vi "Close Manager Refs.vi"(8 "error in (no error)":errorcluster, 11 "teststand-api in":refnum<class "teststand-api.lvclass">) -> (0 "error out":errorcluster, 3 "teststand-api out":refnum<class "teststand-api.lvclass">)   [LabVIEW 2014, in "teststand-api.lvlib" / "teststand-api.lvclass"]
uses:
  teststand-api.lvclass
  teststand-api.lvclass/teststand-api.ctl
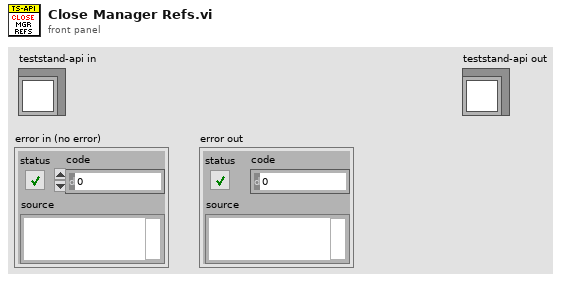
[diagram p1: front panel]
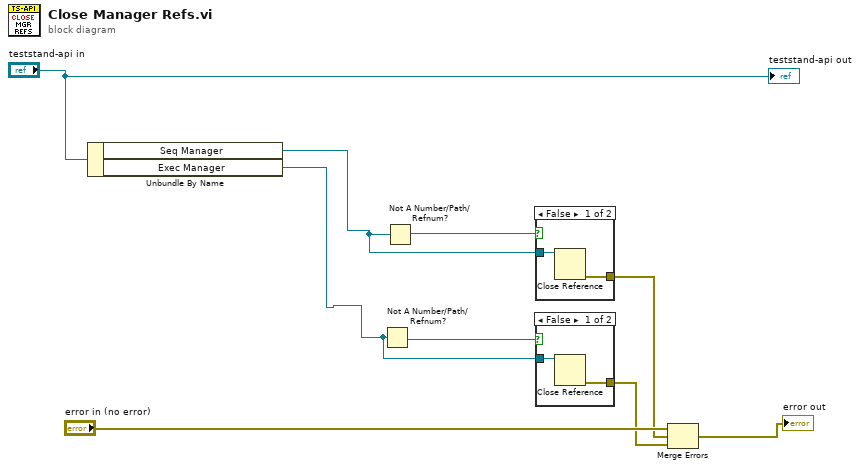
[diagram p0: block diagram]
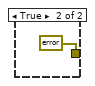
[diagram p2: hidden frame]
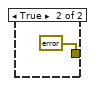
[diagram p3: hidden frame]
diagram:
  n1 = Unbundle By Name("teststand-api in") -> ("Seq Manager"=w5:refnum<k7>, "Exec Manager"=w3:refnum<k7>)
  n2 = Not A Number/Path/Refnum?(number/path/refnum=w3) -> (NaN/Path/Refnum?=w4:bool)
  n3 = Not A Number/Path/Refnum?(number/path/refnum=w5) -> (NaN/Path/Refnum?=w6:bool)
  n4 = case shown="False" w6 {
    tunnel: [w11 errorcluster {"status"=FALSE, "code"=0, "source"=""} ("error out")] -> w2
    tunnel: w5 -> [w10 _]
    frame False {
      n5 = Close Reference(reference=w10) -> (error out=w11:errorcluster)  [unwired: 1 in]
    }
    frame True {
    }
  }
  n6 = case shown="False" w4 {
    tunnel: [w14 errorcluster {"status"=FALSE, "code"=0, "source"=""} ("error out")] -> w1
    tunnel: w3 -> [w13 _]
    frame False {
      n7 = Close Reference(reference=w13) -> (error out=w14:errorcluster)  [unwired: 1 in]
    }
    frame True {
    }
  }
  n8 = Merge Errors("error in (no error)", w2, w1) -> (→"error out":errorcluster)
  "teststand-api out" <- "teststand-api in"
